vi "test_Set-Get Protocol TCP.vi"(8 "error in (no error)":errorcluster, 11 "TestCase in":refnum<class "Instrument Addon Scripting API Custom Device Unit Tests.lvclass">) -> (0 "error out":errorcluster, 3 "TestCase out":refnum<class "Instrument Addon Scripting API Custom Device Unit Tests.lvclass">)   [LabVIEW 2020, in "Instrument Addon Scripting API Custom Device Unit Tests.lvclass"]
uses:
  Instrument Addon Scripting API Custom Device Unit Tests.lvclass
  Includes/Protocols.lvlibp/TCP/TCP.lvclass
  C:/Users/nitest/Desktop/Git 2020/niveristand-instrument-addon-custom-device/Includes/Protocols.lvlibp/Protocol Parent/Protocol Parent.lvclass
  Includes/Protocols.lvlibp/AK RS-xxx/AK RS-xxx.lvclass
  Instrument Addon Scripting API Custom Device Unit Tests.lvclass/Instrument Addon Scripting API Custom Device Unit Tests.ctl
  Includes/Protocols.lvlibp/TCP/Data Access/Write IP Address.vi
  Includes/Protocols.lvlibp/TCP/Data Access/Write Port.vi
  <vilib>/addons/_JKI Toolkits/VI Tester/TestCase.llb/TestCase.lvclass
  APIs/Scripting API/Instrument Addon Scripting API.lvlib
  C:/Program Files (x86)/National Instruments/LabVIEW 2020/vi.lib/addons/_JKI Toolkits/VI Tester/TestCase.llb/TestCase.lvclass
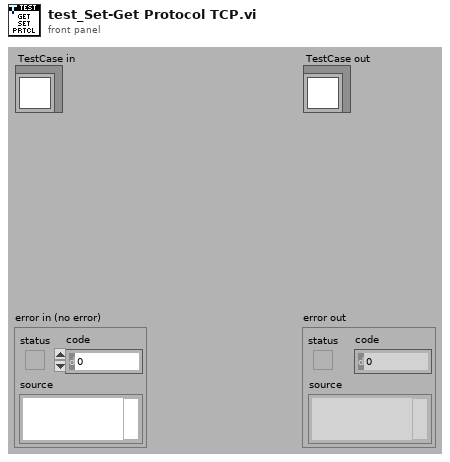
[diagram p1: front panel]
types:
  T1 = typedef "Custom Device API.lvlib/Custom Device Item Ref.ctl" = u64
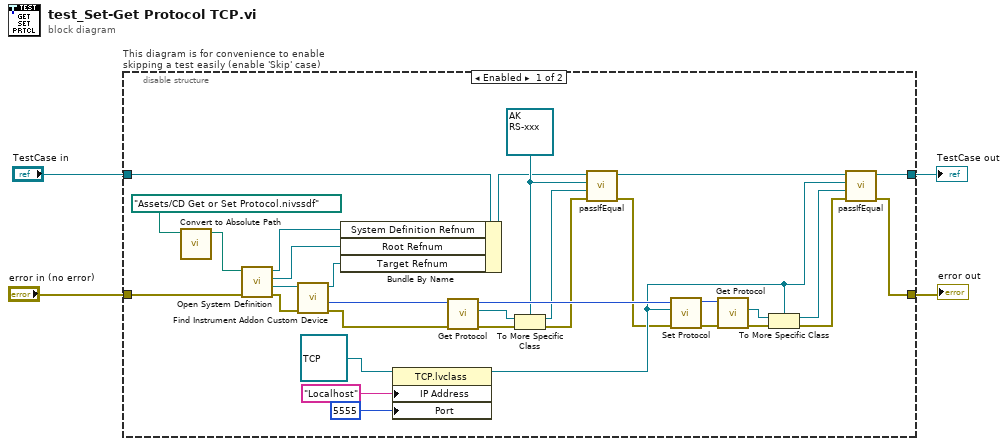
[diagram p0: block diagram]
diagram:
  n1 = disable-structure "This diagram is for convenience to enable skipping a test easily (enable 'Skip' case)" shown="Enabled" {
    disable-tunnel: "TestCase in" -> [w9 w40]
    disable-tunnel: [w26 w38] -> w1
    disable-tunnel: [w24 w39] -> w3
    disable-tunnel: "error in (no error)" -> [w36 w37]
    frame Enabled {
      w14 = refnum<class "AK RS-xxx.lvclass"> refnum ("reference out")
      n2 = call "Convert to Absolute Path.vi"("System Definition File"=path "Assets/CD Get or Set Protocol.nivssdf" ("SDF file")) -> ("Absolute Path"=w34:path)  [unwired: 10 in]
      n3 = call "Open System Definition.vi"("error in (no error)"=w36, "System Definition File"=w34) -> ("error out"=w33:errorcluster, "Target Refnum"=w32:refnum<k24>, "Root Refnum"=w6:refnum<k24>, "System Definition Refnum"=w7:refnum<k24>)  [unwired: 6 in]
      n4 = call "Find Instrument Addon Custom Device.vi"("error in"=w33, "target in"=w32) -> ("error out"=w15:errorcluster, "NodeID"=w19:u64, "target out"=w5:refnum<k24>)  [unwired: 7 in]
      n5 = Bundle By Name(cluster=w9, "System Definition Refnum"=w7, "Root Refnum"=w6, "Target Refnum"=w5) -> (w8:refnum<class "Instrument Addon Scripting API Custom Device Unit Tests.lvclass">)
      n6 = property class="TCP.lvclass"(reference=refnum<class "TCP.lvclass"> refnum ("Protocols.lvlibp:TCP.lvclass"), "IP Address"="Localhost" ("VISA Resource"), "Port"=u16 5555 ("Local Port")) -> (reference out=w17:refnum<class "TCP.lvclass">)  [unwired: 1 in, 1 out]
      n7 = call "Get Protocol.vi"("error in (no error)"=w15, "instrument addon refnum in"=w19) -> ("error out"=w16:errorcluster, "protocol"=w20:refnum<class "Protocol Parent.lvclass">, "instrument addon refnum out"=w18:T1)  [unwired: 7 in]
      n8 = To More Specific Class(target class=w14, reference=w20, error in=w16) -> (specific class reference=w13:refnum<class "AK RS-xxx.lvclass">, error out=w12:errorcluster)
      n9 = call-dynamic "passIfEqual.vi"("error in (no error)"=w12, "y"=w13, "x"=w14, "TestCase in"=w8) -> ("error out"=w10:errorcluster, "TestCase out"=w11:refnum<class "Instrument Addon Scripting API Custom Device Unit Tests.lvclass">)  [unwired: 6 in]
      n10 = call "Set Protocol.vi"("error in (no error)"=w10, "protocol"=w17, "instrument addon refnum in"=w18) -> ("error out"=w30:errorcluster, "instrument addon refnum out"=w31:T1)  [unwired: 7 in]
      n11 = call "Get Protocol.vi"("error in (no error)"=w30, "instrument addon refnum in"=w31) -> ("error out"=w28:errorcluster, "protocol"=w29:refnum<class "Protocol Parent.lvclass">)  [unwired: 7 in, 1 out]
      n12 = To More Specific Class(target class=w17, reference=w29, error in=w28) -> (specific class reference=w25:refnum<class "TCP.lvclass">, error out=w27:errorcluster)
      n13 = call-dynamic "passIfEqual.vi"("error in (no error)"=w27, "y"=w25, "x"=w17, "TestCase in"=w11) -> ("error out"=w24:errorcluster, "TestCase out"=w26:refnum<class "Instrument Addon Scripting API Custom Device Unit Tests.lvclass">)  [unwired: 6 in]
    }
    frame Disabled {
      # "skip test result while test is under development"
      n14 = call <vilib>:"skip.vi"("error in (no error)"=w37, "TestCase in"=w40) -> ("error out"=w39:errorcluster, "TestCase out"=w38:refnum<class "Instrument Addon Scripting API Custom Device Unit Tests.lvclass">)  [unwired: 8 in]
    }
  }
  "error out" <- w3
  "TestCase out" <- w1
